vi "NewDocument__slk_msxml.vi"(11 "error in (no error)":errorcluster) -> (4 "document out":refnum<class "msxml document.lvclass">, 15 "error out":errorcluster)   [LabVIEW 2020, in "MSXML.lvlib" / "msxml document.lvclass"]
doc: "Creates a new MSXML Document object."
uses:
  msxml document.lvclass
  msxml document.lvclass/msxml document.ctl
panel:
  # "NewDocument__slk_msxml.vi\n\nCreates a new MSXML Document object.\n\nNOTICE -- YOU MUST LEAVE THIS NOTICE IN PLACE.\n\nCopyright (c) 2004-2010 Shawn Liu <shawn.liu.cn@gmail.com>\n\nAll rights reserved."
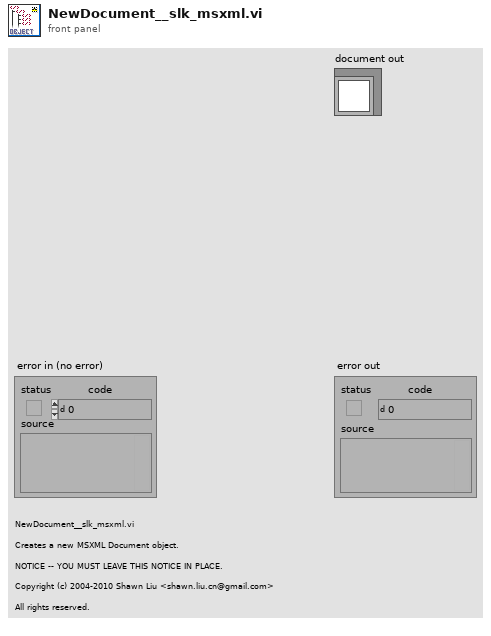
[diagram p1: front panel]
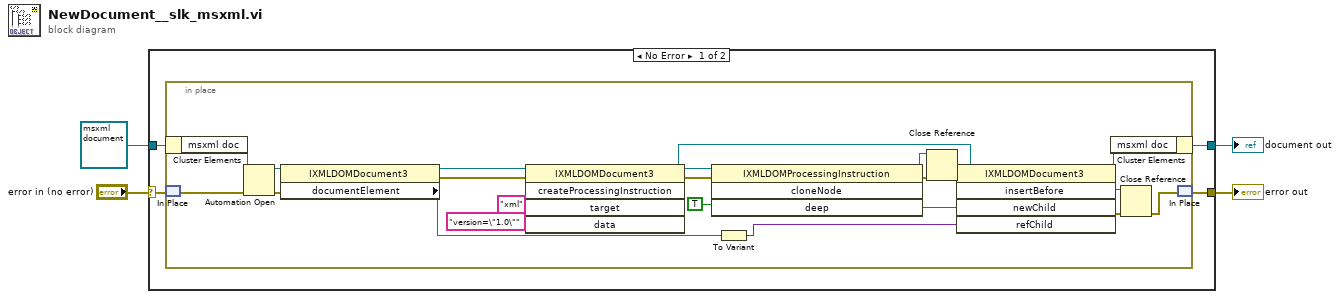
[diagram p0: block diagram]
diagram:
  n1 = case shown="No Error" "error in (no error)" {
    selector: "error in (no error)" -> [w7 w31]
    tunnel: [w5 w32] -> w3
    tunnel: refnum<class "msxml document.lvclass"> refnum ("MSXML in") -> [w8 w32]
    tunnel: [w6 w31] -> w1
    frame No Error {
      n2 = in-place {
        n3 = in-place-cluster #1(w8) -> ("msxml doc"=w12:refnum<k7>)
        n4 = in-place-match #2(w7) -> (w10:errorcluster)
        n5 = Automation Open(error in (no error)=w10, Automation Refnum=w12) -> (Automation Refnum=w30:refnum<k7>, error out=w29:errorcluster)  [unwired: 2 in]
        n6 = property class="IXMLDOMDocument3"(reference=w30, error in=w29) -> (reference out=w28:refnum<k7>, error out=w25:errorcluster, "documentElement"=w17:refnum<k7>)
        n7 = invoke class="IXMLDOMDocument3" method="createProcessingInstruction"(reference=w28, error in=w25, "target"="xml", "data"="version=\"1.0\"") -> (reference out=w15:refnum<k7>, error out=w24:errorcluster, "createProcessingInstruction"=w23:refnum<k7>)  [unwired: 1 in, 2 out]
        n8 = invoke class="IXMLDOMProcessingInstruction" method="cloneNode"(reference=w23, error in=w24, "deep"=TRUE) -> (reference out=w20:refnum<k7>, error out=w21:errorcluster, "cloneNode"=w18:refnum<k7>)  [unwired: 1 in, 1 out]
        n9 = To Variant(anything=w17) -> (Variant=w16:variant)
        n10 = Close Reference(reference=w20, error in (no error)=w21) -> (error out=w19:errorcluster)
        n11 = invoke class="IXMLDOMDocument3" method="insertBefore"(reference=w15, error in=w19, "newChild"=w18, "refChild"=w16) -> (reference out=w11:refnum<k7>, error out=w13:errorcluster, "insertBefore"=w14:refnum<k7>)  [unwired: 1 in, 2 out]
        n12 = in-place-cluster #1("msxml doc"=w11) -> (w5:refnum<class "msxml document.lvclass">)
        n13 = Close Reference(reference=w14, error in (no error)=w13) -> (error out=w9:errorcluster)
        n14 = in-place-match #2(w9) -> (w6:errorcluster)
      }
    }
    frame Error {
    }
  }
  "document out" <- w3
  "error out" <- w1
